vi "Get Value.vi"(8 "error in (no error)":errorcluster, 11 "Protocol in":refnum<class "Protocol.lvclass">) -> (0 "error out":errorcluster, 1 "Movie Series":T1={"Fields"=1, "Lanes"=1, "Acquisition type"=enum."Movie series", "Sweeps"=[]}, 2 "Movie Settings":T5={"Camera Settings"={"Exposure Time (ms)"=100.0, "Binning"=enum."2x2", "Scan Mode"=0, "Frames to Acquire"=1000.0, "Pixel Correction"=FALSE, "Frames to Skip"=0, "File Path"=path "", "Duty cycle"=0.0, "ALEX"=FALSE, "Shutter Enable"=[], "fluidics trigger, ms (0=disabled)"=0.0, "Bit Depth"=0, "Image Width (px)"=0, "Image Height (px)"=0, "Horizontal Offset (px)"=0, "Vertical Offset (px)"=0}, "Auto-Advance"=TRUE, "Auto Focus"=TRUE, "Injection Countdown"=TRUE, "Laser Power (mW)"=0, "Termination Criteria"={"Particle Count Threshold"=0, "Min Frames"=0}} {"Camera Settings"."Exposure Time (ms)" min=1.0 max=10000.0 step=1.0}, 3 "Protocol out":refnum<class "Protocol.lvclass">)   [LabVIEW 2023, in "Automation.lvlib" / "Protocol.lvclass"]
uses:
  Protocol.lvclass
  Resources/Type Defs/Movie Settings.ctl
  Resources/Type Defs/Camera Settings.ctl
  Resources/Type Defs/Movie Series.ctl
  Resources/Type Defs/Movie auto-numbering.ctl
  Resources/Type Defs/Param Sweep.ctl
  Resources/Type Defs/Sweep Parameter.ctl
  Protocol.lvclass/Protocol.ctl
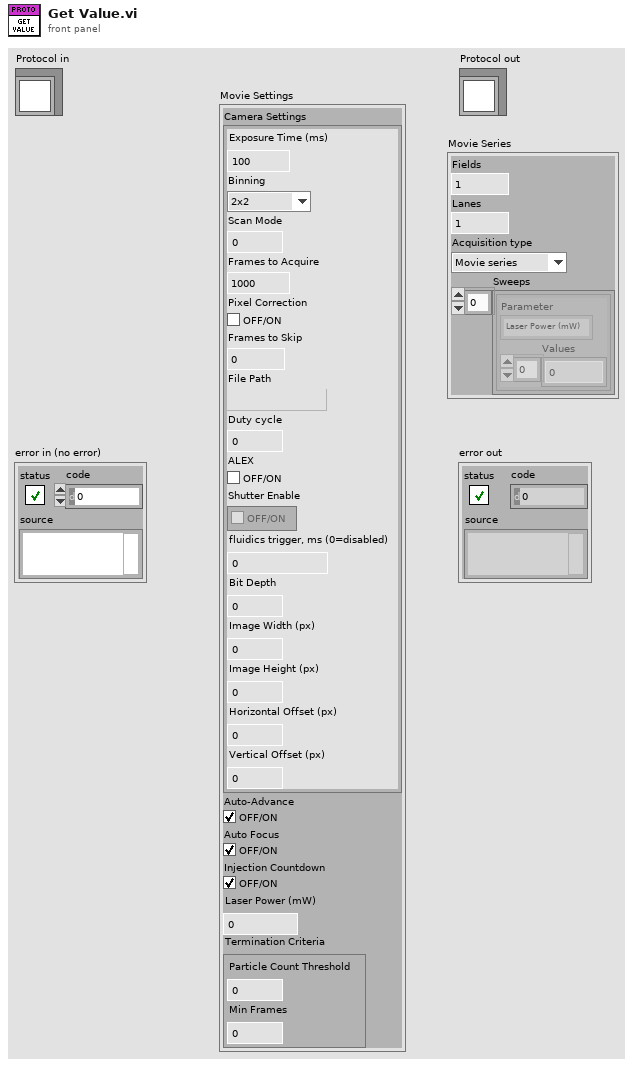
[diagram p1: front panel]
types:
  T1 = typedef "Movie Series.ctl" = cluster{"Fields":i32, "Lanes":i32, "Acquisition type":T2, "Sweeps":T3[]}
  T2 = typedef "Movie auto-numbering.ctl" = enum16{"Single movie", "Movie series", "Multi-lane series", "Sweep Parameter"}
  T3 = typedef "Param Sweep.ctl" = cluster{"Parameter":T4, "Values":u32[]}
  T4 = typedef "Sweep Parameter.ctl" = enum16{"Laser Power (mW)", "Exposure Time (ms)", "Number of Frames", "Laser Line (1,2,3,4)"}
  T5 = typedef "Movie Settings.ctl" = cluster{"Camera Settings":T6, "Auto-Advance":bool, "Auto Focus":bool, "Injection Countdown":bool, "Laser Power (mW)":u32, "Termination Criteria":cluster{"Particle Count Threshold":i32, "Min Frames":i32}}
  T6 = typedef "Camera Settings.ctl" = cluster{"Exposure Time (ms)":dbl, "Binning":enum16{"1x1", "2x2", "4x4"}, "Scan Mode":i32, "Frames to Acquire":dbl, "Pixel Correction":bool, "Frames to Skip":u32, "File Path":path, "Duty cycle":dbl, "ALEX":bool, "Shutter Enable":bool[], "fluidics trigger, ms (0=disabled)":dbl, "Bit Depth":u16, "Image Width (px)":u16, "Image Height (px)":u16, "Horizontal Offset (px)":u16, "Vertical Offset (px)":u16}
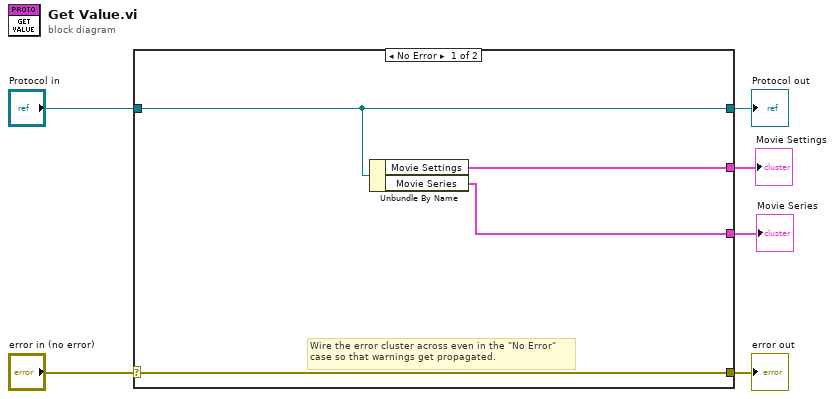
[diagram p0: block diagram]
diagram:
  n1 = case shown="No Error" "error in (no error)" {
    selector: "error in (no error)" -> [w10 w12]
    tunnel: [w10 w12] -> w5
    tunnel: [w9 w11] -> w3
    tunnel: "Protocol in" -> [w9 w11]
    tunnel: [w8 _] -> w2
    tunnel: [w7 _] -> w1
    frame No Error {
      # "Wire the error cluster across even in the \"No Error\"\ncase so that warnings get propagated."
      n2 = Unbundle By Name(w9) -> ("Movie Settings"=w8:T5, "Movie Series"=w7:T1)
    }
    frame Error {
    }
  }
  "error out" <- w5
  "Protocol out" <- w3
  "Movie Settings" <- w2
  "Movie Series" <- w1
